vi "Get Server State Ref.vi"(11 "OOP Query Server in":refnum<class "OOP Query Server.lvclass">) -> (2 "Server State Ref":refnum<data-value>, 3 "OOP Query Server out":refnum<class "OOP Query Server.lvclass">)   [LabVIEW 2019, in "OOP Query Server.lvlib" / "OOP Query Server.lvclass"]
uses:
  OOP Query Server.lvclass
  typeDefs/Server State Data.ctl
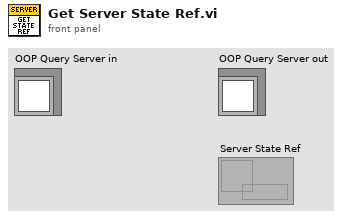
[diagram p1: front panel]
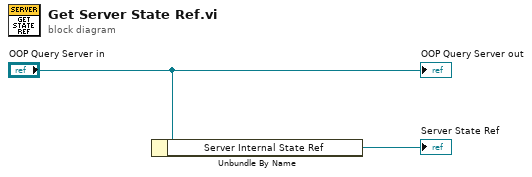
[diagram p0: block diagram]
diagram:
  n1 = Unbundle By Name("OOP Query Server in") -> ("Server Internal State Ref"=→"Server State Ref":refnum<data-value>)
  "OOP Query Server out" <- "OOP Query Server in"
